vi "Hatch Detect.vi"(7 "error in":errorcluster) -> (27 "error out":errorcluster)   [LabVIEW 2018]
uses:
  <vilib>/vision/driver/IMAQdx.llb/IMAQdx Camera Control Mode.ctl
  <vilib>/userdefined/High Color/IMAQdx.ctl
  <vilib>/vision/NI_Vision_Development_Module.lvlib
  <vilib>/vision/driver/NI_Vision_Acquisition_Software.lvlib
  <resource>/objmgr/imaqdx.rc
panel:
  out "Image Out 3":T1(plugin-control)
  out "Image Out 2":T1(plugin-control)
  in  "stop":bool
  out "Image Out":T1(plugin-control)
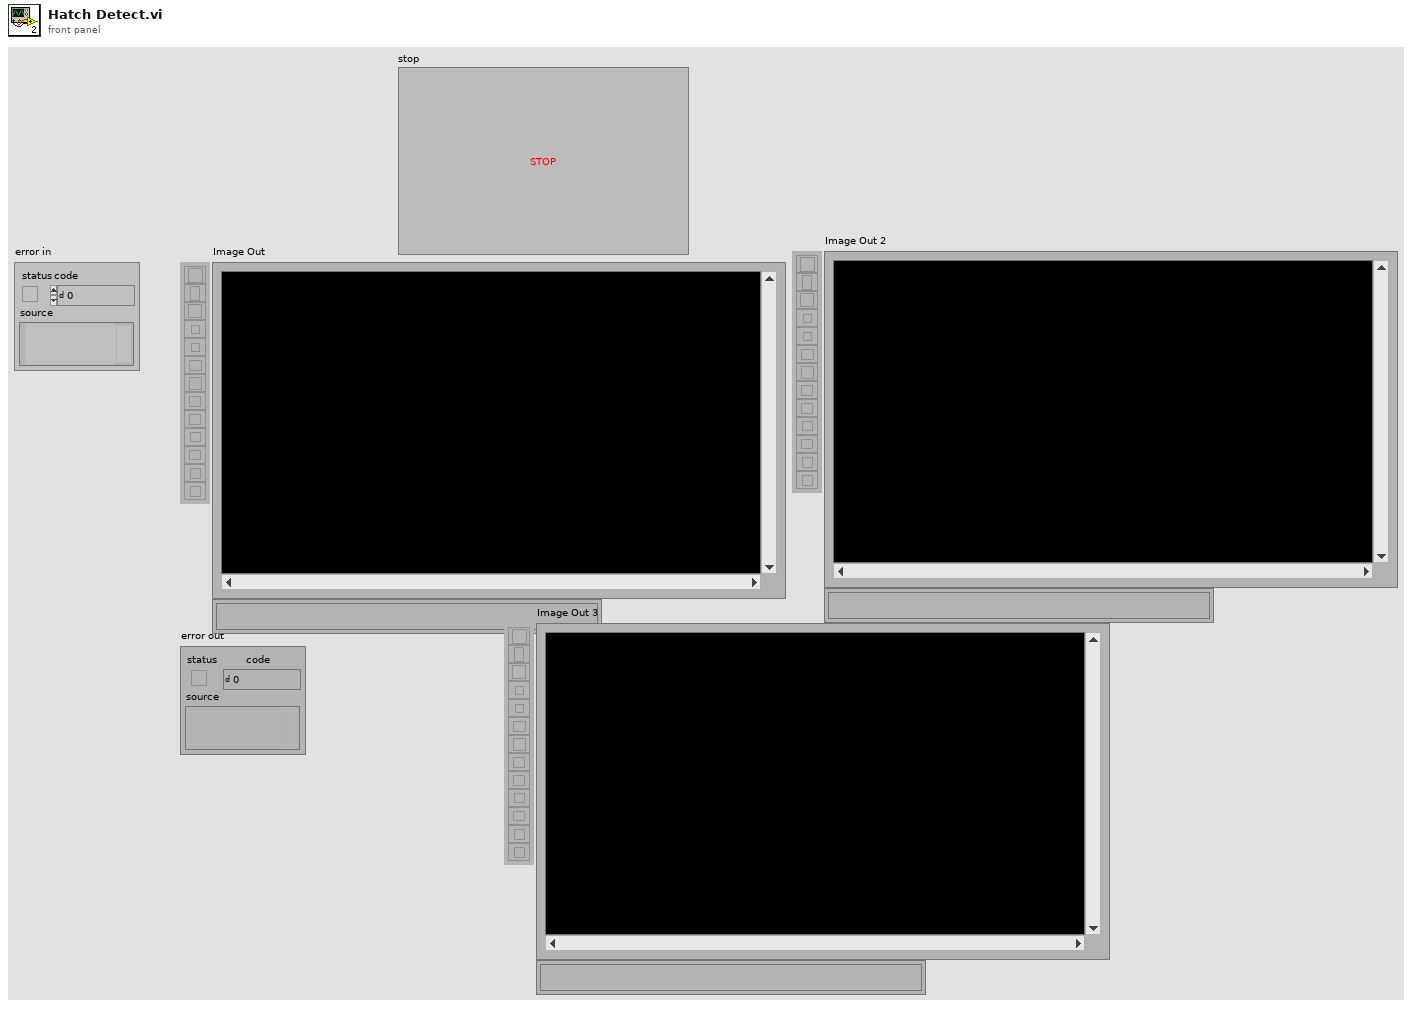
[diagram p1: front panel]
types:
  T1 = typedef "IMAQ Image.ctl" = refnum<image>
  T2 = typedef "Image Type" = u32
  T3 = typedef "IMAQdx.ctl" = refnum<k21>
  T4 = typedef "NI_Vision_Acquisition_Software.lvlib/IMAQdx Camera Control Mode.ctl" = enum32{"Controller", "Listener"}
  T5 = cluster{"Measurement Parameter":i32, "Range Lower Value":dbl, "Range Upper Value":dbl, "Range":bool, "Measurement Type":bool}[]
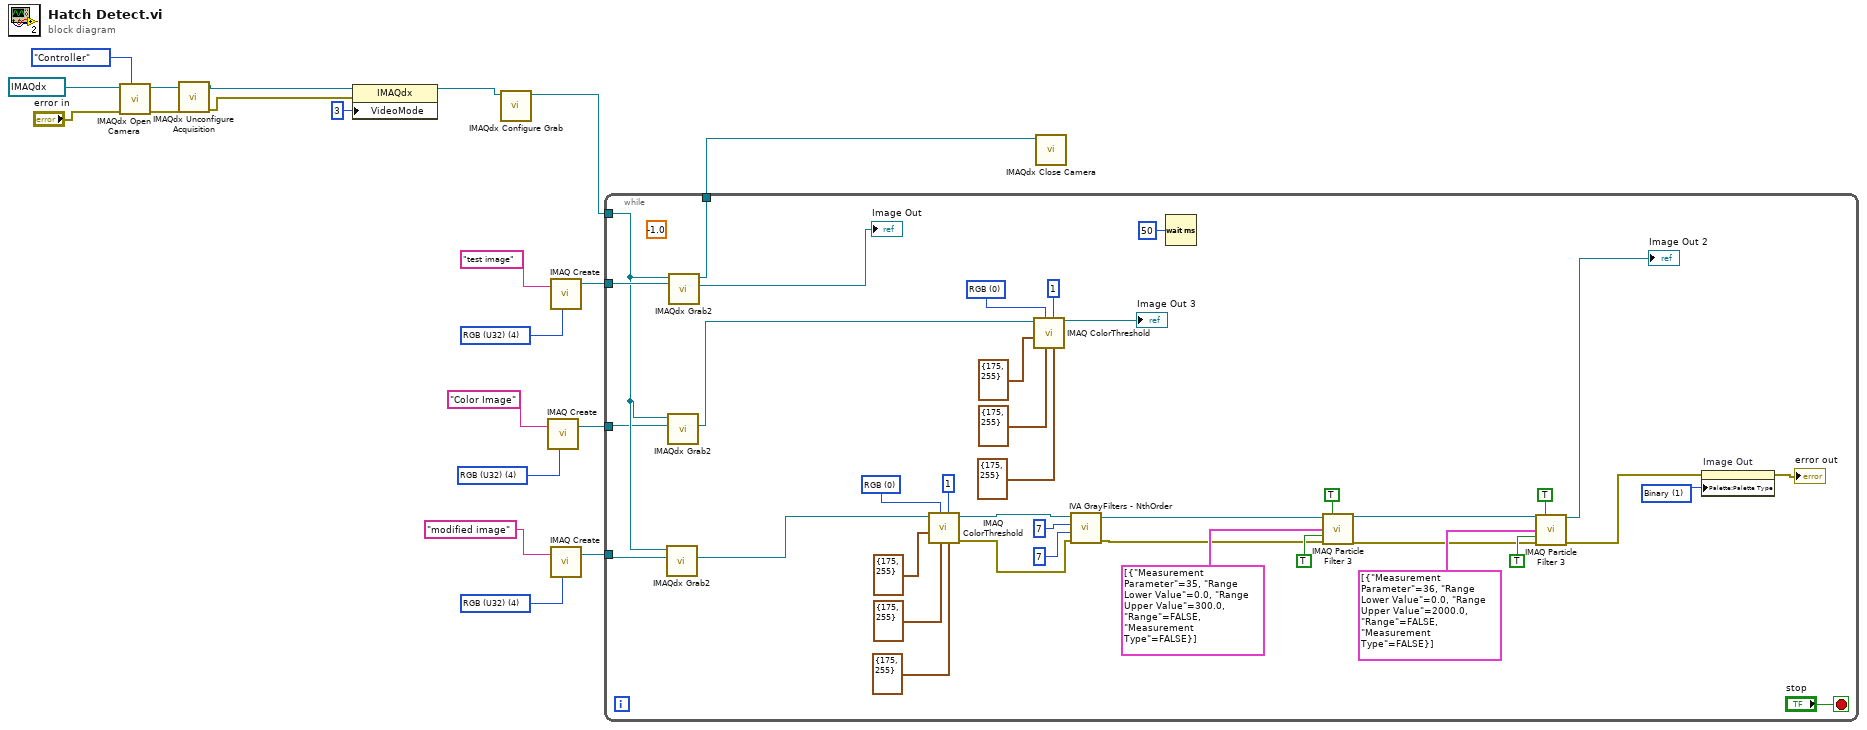
[diagram p0: block diagram]
diagram:
  w2 = T2 4 items=["Grayscale (U8)", "Grayscale (I16)", "Grayscale (SGL)", "Complex (CSG)", "RGB (U32)", "HSL (U32)", "RGB (U64)", "Grayscale (U16)"] ("Image Type")
  w13 = T2 4 items=["Grayscale (U8)", "Grayscale (I16)", "Grayscale (SGL)", "Complex (CSG)", "RGB (U32)", "HSL (U32)", "RGB (U64)", "Grayscale (U16)"] ("Image Type")
  w20 = T2 4 items=["Grayscale (U8)", "Grayscale (I16)", "Grayscale (SGL)", "Complex (CSG)", "RGB (U32)", "HSL (U32)", "RGB (U64)", "Grayscale (U16)"] ("Image Type")
  n1 = call <vilib>:"IMAQdx Open Camera.vi"("Camera Control Mode"=IMAQdx_Camera_Control_Mode."Controller", "error in"="error in", "Session In"=T3 "cam1") -> ("error out"=w7:errorcluster, "Session Out"=w6:T3)  [unwired: 7 in]
  n2 = call <vilib>:"IMAQdx Unconfigure Acquisition.vi"("error in"=w7, "Session In"=w6) -> ("error out"=w4:errorcluster, "Session Out"=w5:T3)  [unwired: 8 in]
  n3 = property class="IMAQdx"(reference=w5, error in=w4, "VideoMode"=u32 3) -> (reference out=w9:T3)  [unwired: 1 out]
  n4 = call <vilib>:"IMAQdx Configure Grab.vi"("Session In"=w9) -> ("Session Out"=w8:T3)  [unwired: 9 in, 1 out]
  n5 = call "IMAQ Create"("Image Name"="Color Image", "Image Type"=w2) -> ("New Image"=w1:T1)  [unwired: 2 in, 2 out]
  n6 = call "IMAQ Create"("Image Name"="test image", "Image Type"=w20) -> ("New Image"=w18:T1)  [unwired: 2 in, 2 out]
  n7 = call "IMAQ Create"("Image Name"="modified image", "Image Type"=w13) -> ("New Image"=w12:T1)  [unwired: 2 in, 2 out]
  n8 = while {
    tunnel: w18 -> [w55]
    tunnel: w8 -> [w31]
    tunnel: [w54] -> w16
    tunnel: w12 -> [w48]
    tunnel: w1 -> [w30]
    stop <- "stop" stop-if-true
    w26 = u16 0 items=["RGB", "HSL", "HSV", "HSI"] ("Color Mode")
    (unwired) sgl -1.0 ("Pixel Color")
    w52 = u16 0 items=["RGB", "HSL", "HSV", "HSI"] ("Color Mode")
    w58 = u32 1 items=["Grayscale", "Binary", "Gradient", "Rainbow", "Temperature", "User Defined", "Binary 16 Bit", "Gradient 16 Bit", "Rainbow 16 Bit", "Temperature 16 Bit", "User Defined 16 Bit"] ("Palette Type")
    n9 = call <vilib>:"IMAQdx Grab2.vi"("Image In"=w48, "Session In"=w31) -> ("Image Out"=w21:T1)  [unwired: 6 in, 3 out]
    n10 = call <vilib>:"IMAQdx Grab2.vi"("Image In"=w30, "Session In"=w31) -> ("Image Out"=w23:T1)  [unwired: 6 in, 3 out]
    n11 = call <vilib>:"IMAQdx Grab2.vi"("Image In"=w55, "Session In"=w31) -> ("Image Out"=→"Image Out":T1, "Session Out"=w54:T3)  [unwired: 6 in, 2 out]
    n12 = call "IMAQ ColorThreshold"("Blue or Luma or Val or Inten Range"=cluster{"Lower value":i32, "Upper value":i32} {"Lower value"=175, "Upper value"=255}, "Replace Value"=1, "Green or Sat Range"=cluster{"Lower value":i32, "Upper value":i32} {"Lower value"=175, "Upper value"=255}, "Color Mode"=w52, "Red or Hue Range"=cluster{"Lower value":i32, "Upper value":i32} {"Lower value"=175, "Upper value"=255}, "Image Src"=w21) -> ("error out"=w45:errorcluster, "Image Dst Out"=w46:T1)  [unwired: 2 in, 2 out]
    n13 = call "IMAQ ColorThreshold"("Blue or Luma or Val or Inten Range"=cluster{"Lower value":i32, "Upper value":i32} {"Lower value"=175, "Upper value"=255}, "Replace Value"=1, "Green or Sat Range"=cluster{"Lower value":i32, "Upper value":i32} {"Lower value"=175, "Upper value"=255}, "Color Mode"=w26, "Red or Hue Range"=cluster{"Lower value":i32, "Upper value":i32} {"Lower value"=175, "Upper value"=255}, "Image Src"=w23) -> ("Image Dst Out"=→"Image Out 3":T1)  [unwired: 2 in, 3 out]
    n14 = call <vilib>:"IVA GrayFilters - NthOrder.vi"("error in"=w45, "Filter size Y"=7, "Filter size X"=7, "Image In"=w46) -> ("error out"=w39:errorcluster, "Image Out"=w40:T1)  [unwired: 6 out]
    n15 = Wait (ms)(milliseconds to wait=u32 50) -> ()  [unwired: 1 out]
    n16 = call "IMAQ Particle Filter 3"("Image Src"=w40, "Connectivity 4/8 (8)"=TRUE, "Selection Values"=T5 [{"Measurement Parameter"=35, "Range Lower Value"=0.0, "Range Upper Value"=300.0, "Range"=FALSE, "Measurement Type"=FALSE}], "Keep/Remove Particles (F)"=TRUE ("Keep/Remove Particles"), "error in (no error)"=w39) -> ("Image Dst Out"=w35:T1, "error out"=w34:errorcluster)  [unwired: 4 in, 5 out]
    n17 = call "IMAQ Particle Filter 3"("Image Src"=w35, "Connectivity 4/8 (8)"=TRUE, "Selection Values"=T5 [{"Measurement Parameter"=36, "Range Lower Value"=0.0, "Range Upper Value"=2000.0, "Range"=FALSE, "Measurement Type"=FALSE}], "Keep/Remove Particles (F)"=TRUE ("Keep/Remove Particles"), "error in (no error)"=w34) -> ("Image Dst Out"=→"Image Out 2":T1, "error out"=w32:errorcluster)  [unwired: 4 in, 5 out]
    n18 = property on="Image Out" class="ImageControl"(error in=w32, "Palette:Palette Type"=w58) -> (error out=→"error out":errorcluster)  [unwired: 1 in, 1 out]
  }
  n19 = call <vilib>:"IMAQdx Close Camera.vi"("Session In"=w16) -> ()  [unwired: 10 in, 1 out]
